vi "Alicat LDO FVIR Example.vi"() -> ()   [LabVIEW 2020]
panel:
  in  "Tare Totalizer":bool
  in  "Tare Flow":bool
  out "Error Out":errorcluster
  in  "Error In":errorcluster
  out "Numeric":i32
  in  "stop":bool
  out "String Data":string[][](array[string])
  in  "VISA Refnum in":refnum<visa-resource-name>
  # "PORT 1: = 40 SLPM Meter\nPORT 3: = 100 SLPM Meter"
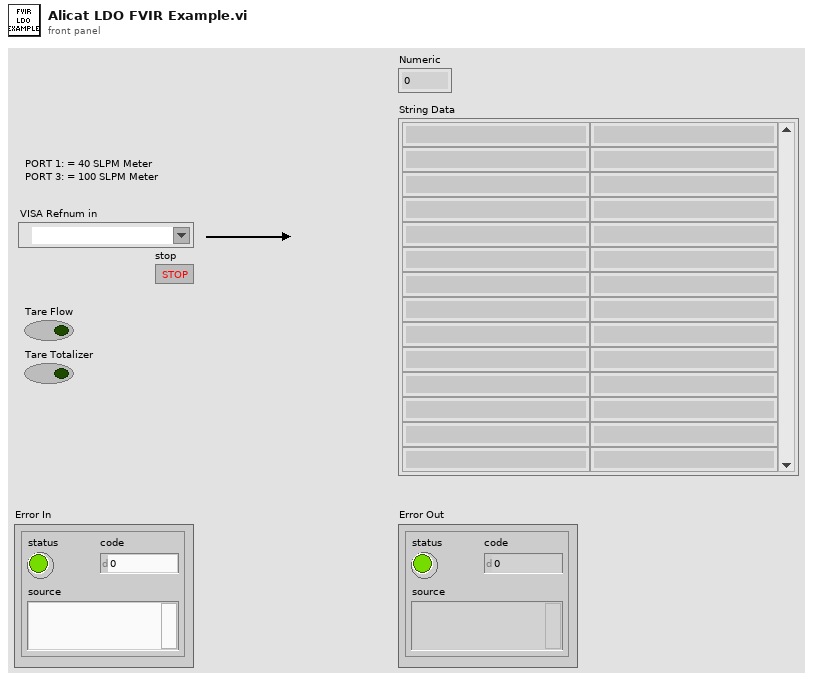
[diagram p1: front panel]
types:
  T1 = typedef "Data Frame.ctl" = cluster{"Absolute Pressure":bool, "Gauge/Diff. Pressure":bool, "Barometric Pressure":bool, "Temperature":bool, "Volumetric":bool, "Mass":bool, "Setpoint":bool, "Valve Drive":bool, "Totalizer":bool, "Totalizer Timer":bool, "Totalizer Average Flow":bool, "Totalizer Peak Flow":bool, "Gas Selected":bool, "Tot. Timer Format":u16}
  T2 = typedef "FMA1600A Units String.ctl" = cluster{"Software Rev":string, "Model Number":string, "Manufacturer Info":string, "Software Sub-Rev":string, "Board Rev":string, "Units of Measure Input":T3}
  T3 = typedef "Units of Measure.ctl" = cluster{"Abs. Pressure":string, "Gauge/Diff. Press.":string, "Barometric Press.":string, "Temperature":string, "Volume":string, "Mass":string, "Setpoint":string, "Valve Drive":string, "Totalizer":string, "Tot. Timer":string, "Tot. Avg. Flow":string, "Tot. Peak Flow":string}
  T4 = cluster{"Absolute Press.":bool, "Gauge/Diff. Press.":bool, "Barometric Press.":bool, "Temperature":bool, "Volumetric":bool, "Mass Flow":bool, "Setpoint":bool, "Valve Drive":bool, "Totalizer":bool, "Tot. Timer [s]":bool, "Tot. Avg. Flow":bool, "Tot. Peak Flow":bool, "Gas Selected":bool, "Log Data":bool}
  T5 = typedef "Data Cluster.ctl" = cluster{"Absolute Pressure":dbl, "Gauge/Diff. Pressure":dbl, "Barometric Pressure":dbl, "Temperature":dbl, "Volumetric Flow":dbl, "Mass Flow":dbl, "Setpoint":dbl, "Valve Drive":dbl, "Totalizer":dbl, "[hr]":dbl, "[min]":dbl, "[sec]":dbl, "Totalizer Average Flow":dbl, "Totalizer Peak Flow":dbl, "Gas selected":string}
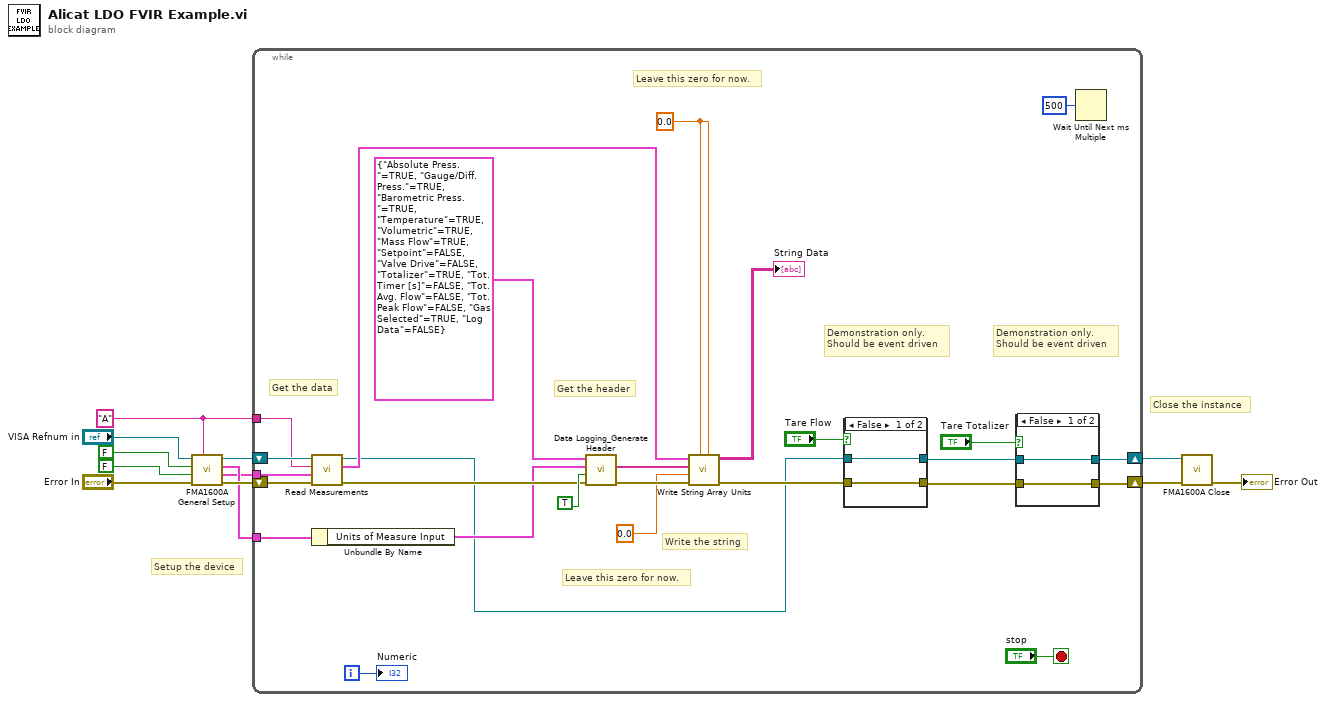
[diagram p0: block diagram]
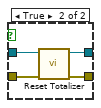
[diagram p2: hidden frame]
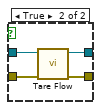
[diagram p3: hidden frame]
diagram:
  w4 = "A" ("Unit ID")
  # "Close the instance"
  # "Setup the device"
  n1 = call "FMA1600A General Setup.vi"("Unit ID"=w4, "error in (no error)"="Error In", "Select Gas?"=FALSE, "Set STP Register"=FALSE, "VISA Refnum in"="VISA Refnum in") -> ("error out"=w9:errorcluster, "Data Frame Format"=w3:T1, "Measurement Units"=w7:T2, "VISA Refnum out"=w8:refnum<visa-resource-name>)  [unwired: 3 in]
  n2 = while {
    tunnel: w7 -> [w33]
    tunnel: w4 -> [w25]
    tunnel: w3 -> [w24]
    shift-right: [w13] -> w6
    shift-left: w9 -> [w38]
    shift-right: [w14] -> w5
    shift-left: w8 -> [w37]
    i -> [w21]
    stop <- "stop" stop-if-true
    w29 = 0.0 ("HHV_1")
    # "Demonstration only. \nShould be event driven"
    # "Demonstration only. \nShould be event driven"
    # "Write the string"
    # "Get the header"
    # "Get the data"
    # "Leave this zero for now."
    # "Leave this zero for now."
    n3 = call "Read Measurements.vi"("error in"=w38, "Data Frame Format In"=w24, "Unit ID (A)"=w25, "VISA Session In"=w37) -> ("error out"=w34:errorcluster, "Data Cluster"=w31:T5, "VISA Session Out"=w16:refnum<visa-resource-name>)  [unwired: 5 out]
    n4 = Unbundle By Name(w33) -> ("Units of Measure Input"=w32:T3)
    n5 = call "Data Logging_Generate Header.vi"("error in"=w34, "Include Units\nin Header (F)"=TRUE ("Include Units\nin Header (default is F)"), "Units of Measure Input"=w32, "Data Logging Options"=T4 {"Absolute Press."=TRUE, "Gauge/Diff. Press."=TRUE, "Barometric Press."=TRUE, "Temperature"=TRUE, "Volumetric"=TRUE, "Mass Flow"=TRUE, "Setpoint"=FALSE, "Valve Drive"=FALSE, "Totalizer"=TRUE, "Tot. Timer [s]"=FALSE, "Tot. Avg. Flow"=FALSE, "Tot. Peak Flow"=FALSE, "Gas Selected"=TRUE, "Log Data"=FALSE}) -> ("error out"=w30:errorcluster, "Header Array"=w28:string[])  [unwired: 5 in, 1 out]
    n6 = call "Write String Array Units.vi"("Total_1"=w29, "HHV_1"=w29, "Error In"=w30, "Gross Heating Value, Vol (Real, Dry)"=0.0, "Header Array"=w28, "Data Cluster"=w31) -> ("Error Out"=w18:errorcluster, "String Data"=→"String Data":string[][])  [unwired: 4 in]
    n7 = case shown="False" "Tare Flow" {
      tunnel: w18 -> [w45 w50]
      tunnel: [w45 w49] -> w17
      tunnel: w16 -> [w46 w48]
      tunnel: [w46 w47] -> w15
      frame False {
      }
      frame True {
        n8 = call "Tare Flow.vi"("error in"=w50, "VISA Session In"=w48) -> ("error out"=w49:errorcluster, "VISA Session Out"=w47:refnum<visa-resource-name>)  [unwired: 8 in]
      }
    }
    n9 = case shown="False" "Tare Totalizer" {
      tunnel: w17 -> [w39 w44]
      tunnel: w15 -> [w40 w43]
      tunnel: [w40 w42] -> w14
      tunnel: [w39 w41] -> w13
      frame False {
      }
      frame True {
        n10 = call "Reset Totalizer.vi"("error in"=w44, "VISA Session In"=w43) -> ("error out"=w41:errorcluster, "VISA Session Out"=w42:refnum<visa-resource-name>)  [unwired: 7 in, 1 out]
      }
    }
    n11 = Wait Until Next ms Multiple(millisecond multiple=u32 500) -> ()  [unwired: 1 out]
    "Numeric" <- w21
  }
  n12 = call "FMA1600A Close.vi"("error in (no error)"=w6, "VISA Refnum in"=w5) -> ("error out"=→"Error Out":errorcluster)  [unwired: 9 in]
